vi "Get Color Table.vi"(8 "错误输入":errorcluster, 9 "Size of Color Table":u8, 10 "Offset In":i32, 11 "Gif data In":string) -> (0 "错误输出":errorcluster, 1 "Color Table":u32[](array[numeric]), 2 "Offset Out":i32, 3 "Gif data Out":string)   [LabVIEW 2012, in "Picture Box Tools.lvlib" / "Gif Image.lvclass"]
uses:
  Gif Image.lvclass
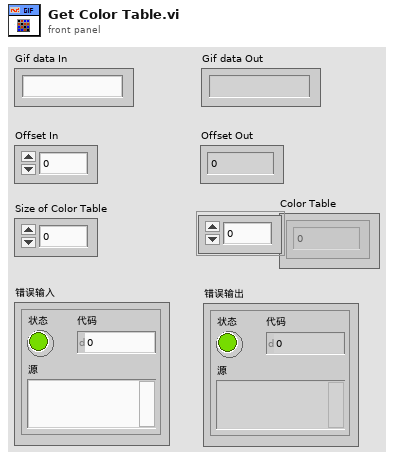
[diagram p1: front panel]
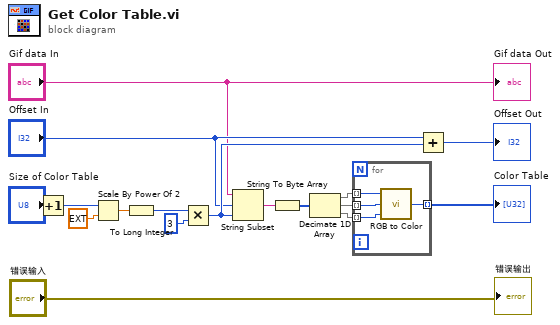
[diagram p0: block diagram]
diagram:
  n1 = Increment(x="Size of Color Table") -> (x+1=w3:u8)
  n2 = Scale By Power Of 2(n=w3, x=ext 1.0) -> (x*2^n=w5:ext)
  n3 = To Long Integer(number=w5) -> (32bit integer=w6:i32)
  n4 = Multiply(x=w6, y=3) -> (x*y=w10:i32)
  n5 = String Subset(string="Gif data In", offset (0)="Offset In", length (rest)=w10) -> (substring=w11:string)
  n6 = String To Byte Array(string=w11) -> (unsigned byte array=w12:u8[])
  n7 = Decimate 1D Array(w12) -> (w13:u8[], w14:u8[], w15:u8[])
  n8 = for {
    tunnel: w13 -> [w21] mode=indexing
    tunnel: w14 -> [w20] mode=indexing
    tunnel: w15 -> [w19] mode=indexing
    tunnel: [w18] -> w17 mode=indexing
    n9 = call <vilib>:"RGB to Color.vi"("B"=w19, "G"=w20, "R"=w21) -> ("Color"=w18:u32)
  }
  "Color Table" <- w17
  n10 = Add(x="Offset In", y=w10) -> (x+y=→"Offset Out":i32)
  "Gif data Out" <- "Gif data In"
  "错误输出" <- "错误输入"
